vi "CycleX.vi"(0 "Devices queue":refnum<queue>, 1 "Program only changes":bool, 5 "Program during MOT loading":bool, 7 "Igor Inform String":string[](array[string]), 9 "Additional wait time (s)":dbl, 11 "error in":errorcluster) -> (8 "error out":errorcluster)   [LabVIEW 2013]
uses:
  DeviceVIs/Device/Device.lvclass
  DeviceVIs/Master Device/Master Device.lvclass
  Globals/Total Time.vi
panel:
  # "Status and timing"
  # "Igor options"
  # "Hardware control"
  # "This option starts the pulse blaster and then programs the external devices.  If the MOT loading time is not long enough for this process to complete there will be problems."
  # "When set, this option only\nasks a device to program\nitself if it's hardware image\nhas actually changed."
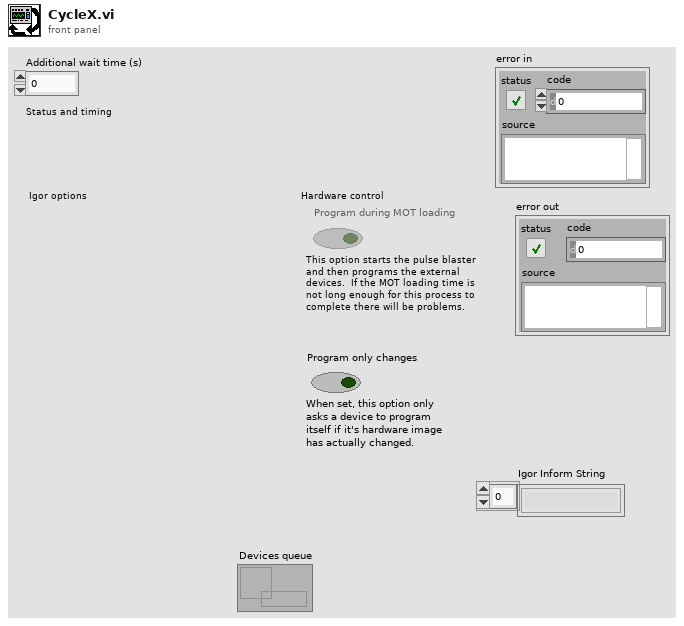
[diagram p1: front panel]
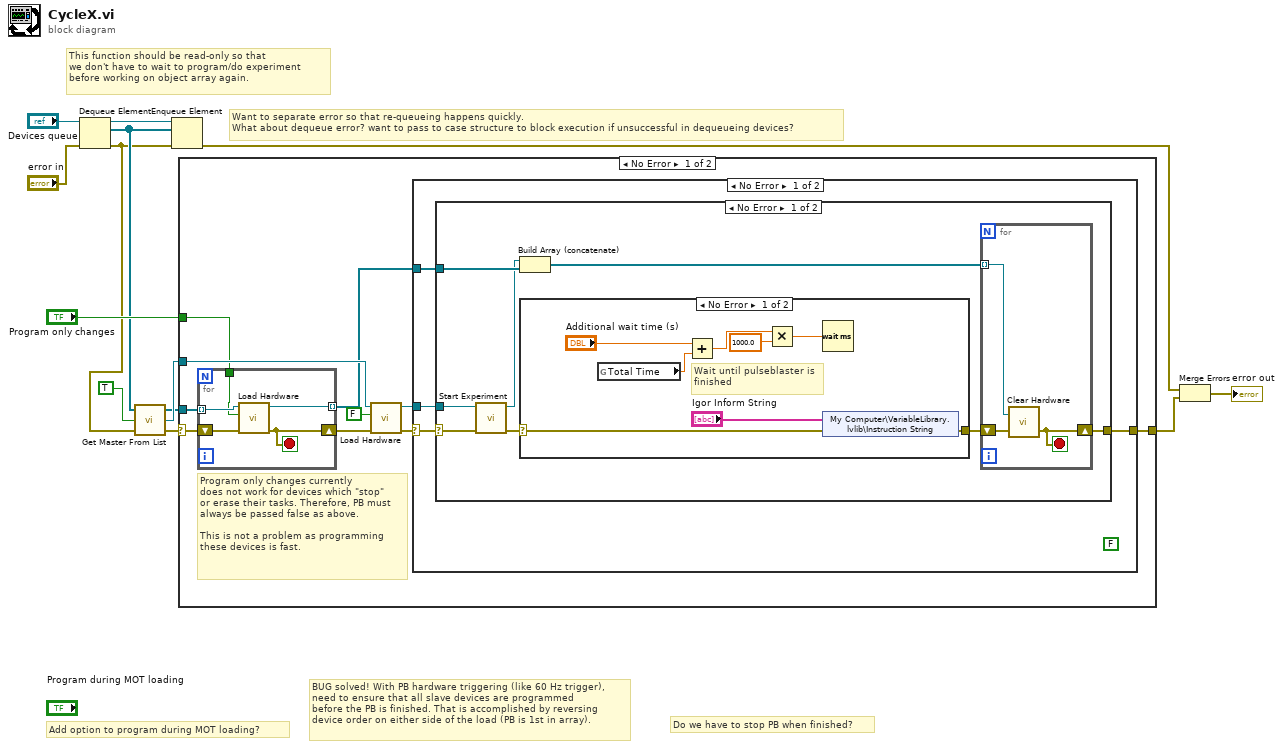
[diagram p0: block diagram]
diagram:
  # "This function should be read-only so that \nwe don't have to wait to program/do experiment \nbefore working on object array again."
  # "Want to separate error so that re-queueing happens quickly.\nWhat about dequeue error? want to pass to case structure to block execution if unsuccessful in dequeueing devices?"
  # "BUG solved! With PB hardware triggering (like 60 Hz trigger),\nneed to ensure that all slave devices are programmed\nbefore the PB is finished. That is accomplished by reversing\ndevice order on either side of the load (PB is 1st in array)."
  # "Do we have to stop PB when finished?"
  # "Add option to program during MOT loading?"
  n1 = Dequeue Element(queue="Devices queue", error in (no error)="error in") -> (queue out=w7:refnum<queue>, element=w6:refnum<class "Device.lvclass">[], error out=w1:errorcluster)  [unwired: 1 in, 1 out]
  n2 = call "Get Master From List.vi"("error in"=w1, "Del From List?"=TRUE, "Device List in"=w6) -> ("error out"=w10:errorcluster, "Master Device"=w12:refnum<class "Master Device.lvclass">, "Device List out"=w11:refnum<class "Device.lvclass">[])
  n3 = Enqueue Element(queue=w7, element=w6, error in (no error)=w1) -> (error out=w3:errorcluster)  [unwired: 1 in, 2 out]
  n4 = case shown="No Error" w10 {
    selector: w10 -> [w18 w55]
    tunnel: w12 -> [w22 _]
    tunnel: w11 -> [w21 _]
    tunnel: [w17 w55] -> w5
    tunnel: "Program only changes" -> [w15 _]
    frame No Error {
      # "Program only changes currently\ndoes not work for devices which \"stop\"\nor erase their tasks. Therefore, PB must\nalways be passed false as above.\n\nThis is not a problem as programming\nthese devices is fast."
      n5 = for {
        tunnel: w21 -> [w54] mode=indexing
        shift-right: [w52] -> w23
        shift-left: w18 -> [w53]
        tunnel: [w51] -> w20 mode=indexing
        tunnel: w15 -> [w50]
        stop <- w52 stop-if-true
        n6 = call-dynamic "Load Hardware.vi"("error in (no error)"=w53, "Program only changes"=w50, "Device in"=w54) -> ("error out"=w52:errorcluster, "Device out"=w51:refnum<class "Device.lvclass">)  [unwired: 7 in]
      }
      n7 = call-dynamic "Load Hardware.vi"("error in (no error)"=w23, "Program only changes"=FALSE, "Master Device in"=w22) -> ("error out"=w16:errorcluster, "Master Device out"=w19:refnum<class "Master Device.lvclass">)  [unwired: 7 in]
      n8 = case shown="No Error" w16 {
        selector: w16 -> [w24 w49]
        tunnel: w20 -> [w25 _]
        tunnel: [w27 w49] -> w17
        tunnel: w19 -> [w26 _]
        frame No Error {
          (unwired) FALSE ("Del From List?")
          n9 = case shown="No Error" w24 {
            selector: w24 -> [w34 w48]
            tunnel: w26 -> [w35 _]
            tunnel: w25 -> [w32 _]
            tunnel: [w33 w48] -> w27
            frame No Error {
              n10 = call-dynamic "Start Experiment.vi"("error in (no error)"=w34, "Master Device in"=w35) -> ("error out"=w31:errorcluster, "Master Device out"=w28:refnum<class "Master Device.lvclass">)  [unwired: 8 in]
              n11 = Build Array (concatenate)(w28, w32) -> (w29:refnum<class "Device.lvclass">[])
              n12 = case shown="No Error" w31 {
                selector: w31 -> [w38 w44]
                tunnel: [w37 w44] -> w30
                frame No Error {
                  # "Wait until pulseblaster is\nfinished"
                  n13 = global read "Total Time.vi" "Total Time"() -> (w42:dbl)
                  n14 = Add(x="Additional wait time (s)", y=w42) -> (x+y=w40:dbl)
                  n15 = Multiply(x=w40, y=1000.0) -> (x*y=w39:dbl)
                  n16 = Wait (ms)(milliseconds to wait=w39) -> ()  [unwired: 1 out]
                  n17 = shared-variable "My Computer\\VariableLibrary.lvlib\\Instruction String"("Igor Inform String", error in=w38) -> (error out=w37:errorcluster)
                }
                frame Error {
                }
              }
              n18 = for {
                shift-right: [w46] -> w33
                shift-left: w30 -> [w47]
                tunnel: w29 -> [w45] mode=indexing
                stop <- w46 stop-if-true
                n19 = call-dynamic "Clear Hardware.vi"("error in (no error)"=w47, "Device in"=w45) -> ("error out"=w46:errorcluster)  [unwired: 1 out]
              }
            }
            frame Error {
            }
          }
        }
        frame Error {
        }
      }
    }
    frame Error {
    }
  }
  n20 = Merge Errors(w3, w5) -> (→"error out":errorcluster)
